vi "RTMain.Initialize.vi"(11 "Device Reference in":T1 format="%.0x") -> (0 "error out":errorcluster, 2 "Name":string, 3 "Parameters":T2 {"Settings"."Data Refs"."Write Refs" format="%.0x"; "Settings"."Data Refs"."Read Refs" format="%.0x"; "Settings"."Write Locations"."DataType" items=["Boolean"=1, "SByte"=2, "Byte"=3, "Int16"=4, "UInt16"=5, "Int32"=6, "UInt32"=7, "Int64"=8, "UInt64"=9, "Float"=10, "Double"=11, "String"=12, "DateTime"=13, "ByteString"=15, "Array of Boolean"=101, "Array of SByte"=102, "Array of Byte"=103, "Array of Int16"=104, "Array of UInt16"=105, "Array of Int32"=106, "Array of UInt32"=107, "Array of Int64"=108, "Array of UInt64"=109, "Array of Float"=110, "Array of Double"=111, "Array of String"=112, "Array of DateTime"=113, "Array of ByteString"=115]; "Settings"."StatusRefs"."Chan Refs" format="%.0x"})   [LabVIEW 2013, in "OPC UA Client Engine.lvlib"]
uses:
  OPC UA Client Engine.lvlib
  Types/PollEngine.Parameters.ctl
  Shared/Compiled.Settings.ctl
  Shared/Connection.Properties.ctl
  Shared/PollEngine.Settings.ctl
  <vilib>/NI Veristand/Custom Device API/Data Reference.ctl
  Shared/WriteData.Info.ctl
  Shared/ReadWriteRefs.ctl
  <vilib>/NI Veristand/Custom Device API/Custom Device Item Ref.ctl
  <vilib>/NI Veristand/Custom Device API/Get Item Property (Variant).vi
  Shared/Constants.vi
  <vilib>/NI Veristand/Custom Device API/Custom Device API.lvlib
  Shared/OPC UA Client Shared.lvlib
  <vilib>/OPCUA/NI OPC UA Client.lvlib
  <vilib>/NI VeriStand/Custom Device Tools/Custom Device Utility Library/Custom Device Utility Library.lvlib
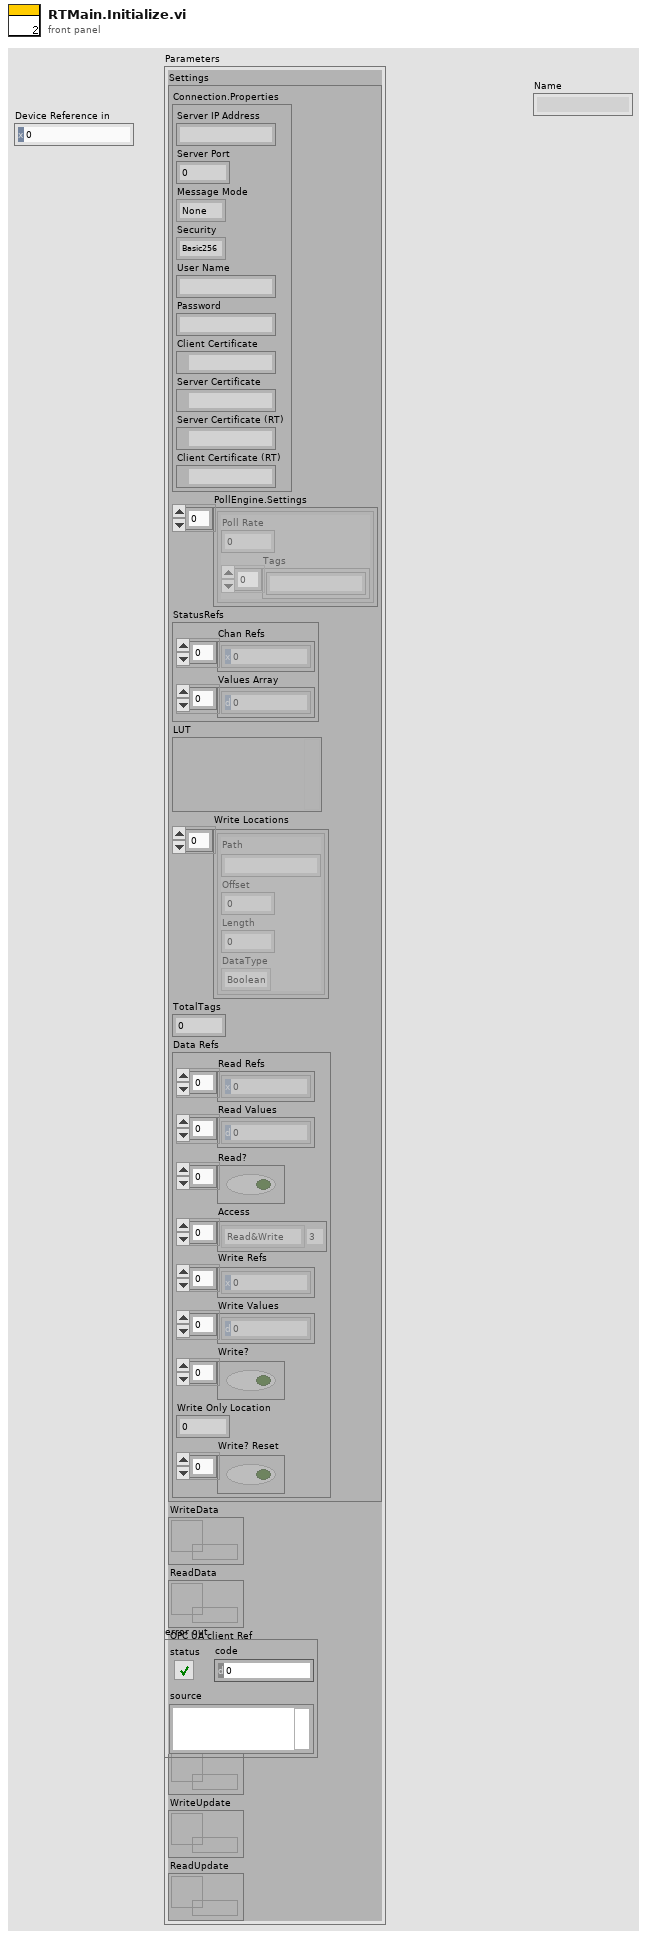
[diagram p1: front panel]
types:
  T1 = typedef "Custom Device API.lvlib/Custom Device Item Ref.ctl" = u64
  T2 = typedef "OPC UA Client Engine.lvlib/PollEngine.Parameters.ctl" = cluster{"Settings":T3, "WriteData":refnum<k33>, "ReadData":refnum<k33>, "OPC UA client Ref":refnum<k21>, "Data Change":refnum<user-event>, "StatusData":refnum<k33>, "WriteUpdate":refnum<k33>, "ReadUpdate":refnum<k33>}
  T3 = typedef "OPC UA Client Shared.lvlib/Compiled.Settings.ctl" = cluster{"Connection.Properties":T4, "PollEngine.Settings":T5[], "StatusRefs":cluster{"Chan Refs":T6[], "Values Array":dbl[]}, "LUT":variant, "Write Locations":T7[], "TotalTags":u32, "Data Refs":T8}
  T4 = typedef "OPC UA Client Shared.lvlib/Connection.Properties.ctl" = cluster{"Server IP Address":string, "Server Port":u16, "Message Mode":enum16{"None", "Sign", "Sign and Encrypt"}, "Security":enum16{"Basic256", "Basic128Rsa15"}, "User Name":string, "Password":string, "Client Certificate":path, "Server Certificate":path, "Server Certificate (RT)":path, "Client Certificate (RT)":path}
  T5 = typedef "OPC UA Client Shared.lvlib/PollEngine.Settings.ctl" = cluster{"Poll Rate":dbl, "Tags":string[]}
  T6 = typedef "Custom Device API.lvlib/Data Reference.ctl" = i32
  T7 = typedef "OPC UA Client Shared.lvlib/WriteData.Info.ctl" = cluster{"Path":string, "Offset":i32, "Length":i32, "DataType":u32}
  T8 = typedef "OPC UA Client Shared.lvlib/ReadWriteRefs.ctl" = cluster{"Read Refs":T6[], "Read Values":dbl[], "Read?":bool[], "Access":enum8{"Null", "Read", "Write", "Read&Write"}[], "Write Refs":T6[], "Write Values":dbl[], "Write?":bool[], "Write Only Location":u32, "Write? Reset":bool[]}
  T9 = cluster{"read mode":enum16{"polling", "blocking"}, "write mode":enum16{"polling", "blocking"}}
  T10 = cluster{"message mode":enum16{"None", "Sign", "Sign and Encrypt"}, "security":enum16{"Basic256", "Basic128Rsa15"}}
  T11 = typedef "Custom Device API.lvlib/Custom Device Item Info.ctl" = cluster{"Name":string, "Is Channel":bool, "GUID":string, "Is Waveform":bool}
  T12 = typedef "Custom Device API.lvlib/Custom Device Target Type.ctl" = enum16{"PharLap", "VxWorks", "Windows"}
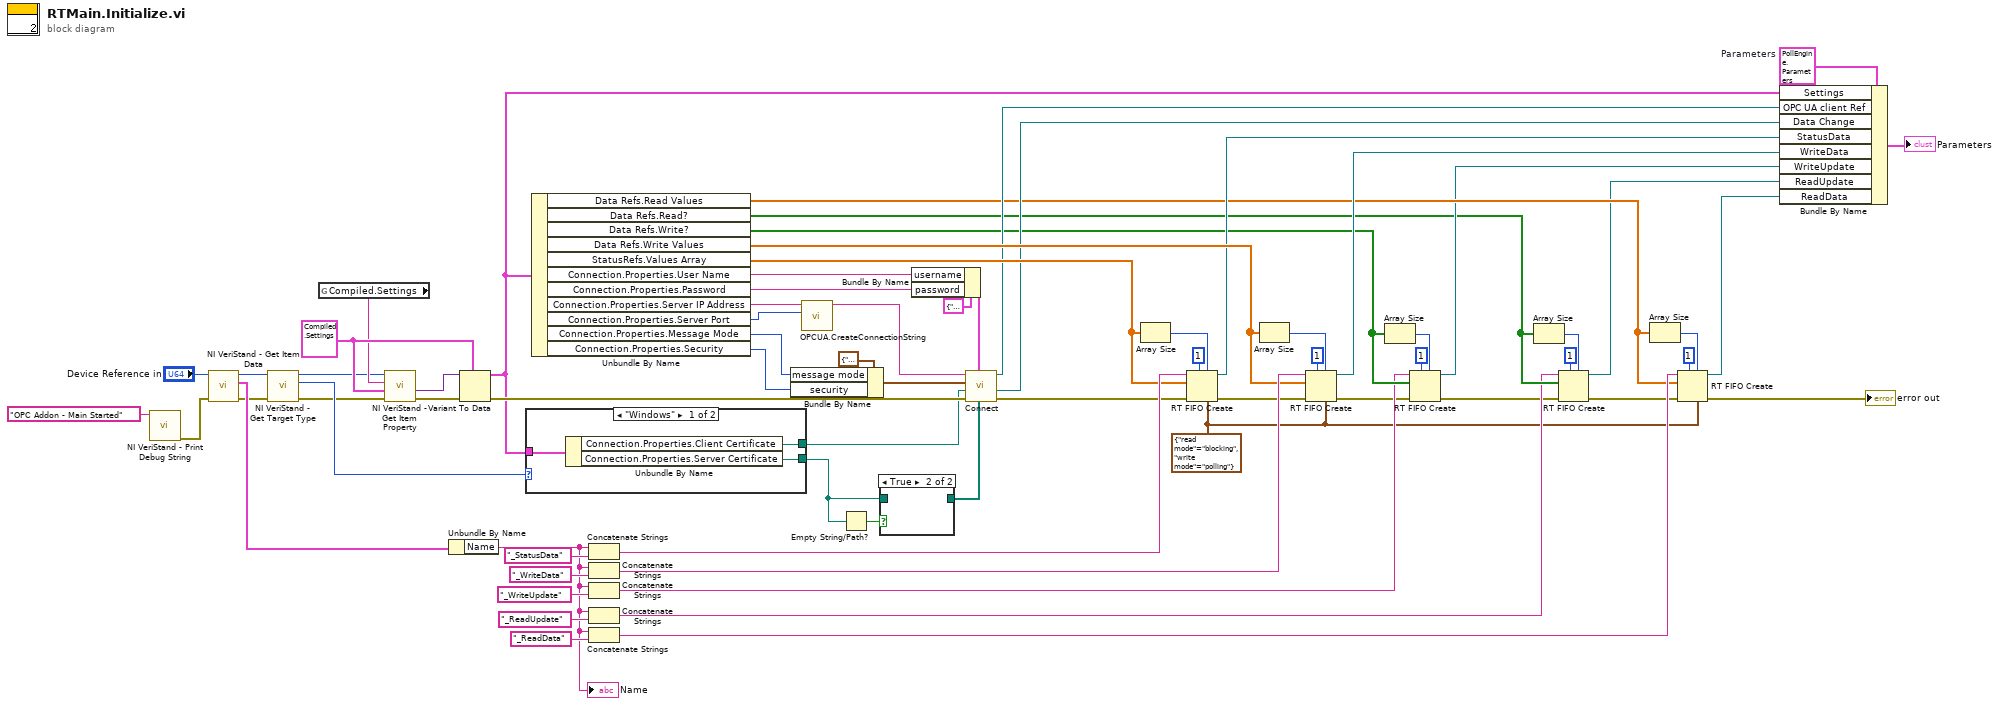
[diagram p0: block diagram]
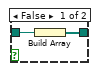
[diagram p2: hidden frame]
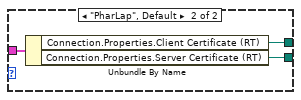
[diagram p3: hidden frame]
diagram:
  w12 = T9 {"read mode"=enum."blocking", "write mode"=enum."polling"} ("r/w modes (polling,polling)")
  w70 = T2 {"Settings"={"Connection.Properties"={"Server IP Address"="", "Server Port"=0, "Message Mode"=enum."None", "Security"=enum."Basic256", "User Name"="", "Password"="", "Client Certificate"=path "", "Server Certificate"=path "", "Server Certificate (RT)"=path "", "Client Certificate (RT)"=path ""}, "PollEngine.Settings"=[], "StatusRefs"={"Chan Refs"=[], "Values Array"=[]}, "LUT"=variant, "Write Locations"=[], "TotalTags"=0, "Data Refs"={"Read Refs"=[], "Read Values"=[], "Read?"=[], "Access"=[], "Write Refs"=[], "Write Values"=[], "Write?"=[], "Write Only Location"=0, "Write? Reset"=[]}}, "WriteData"=refnum, "ReadData"=refnum, "OPC UA client Ref"="", "Data Change"=refnum, "StatusData"=refnum, "WriteUpdate"=refnum, "ReadUpdate"=refnum}  # Parameters
  w63 = T3 {"Connection.Properties"={"Server IP Address"="", "Server Port"=0, "Message Mode"=enum."None", "Security"=enum."Basic256", "User Name"="", "Password"="", "Client Certificate"=path "", "Server Certificate"=path "", "Server Certificate (RT)"=path "", "Client Certificate (RT)"=path ""}, "PollEngine.Settings"=[], "StatusRefs"={"Chan Refs"=[], "Values Array"=[]}, "LUT"=variant, "Write Locations"=[], "TotalTags"=0, "Data Refs"={"Read Refs"=[], "Read Values"=[], "Read?"=[], "Access"=[], "Write Refs"=[], "Write Values"=[], "Write?"=[], "Write Only Location"=0, "Write? Reset"=[]}} ("Compiled.Settings")
  n1 = call <vilib>:"NI VeriStand - Print Debug String.vi"("Message"="OPC Addon - Main Started") -> ("error out"=w25:errorcluster)  [unwired: 10 in]
  n2 = call <vilib>:"NI VeriStand - Get Item Data.vi"("error in (no error)"=w25, "Item Ref in"="Device Reference in") -> ("error out"=w2:errorcluster, "Item Info"=w64:T11, "Item Ref out"=w1:T1)  [unwired: 6 in, 1 out]
  n3 = call <vilib>:"NI VeriStand - Get Target Type.vi"("error in (no error)"=w2, "Item Ref in"=w1) -> ("error out"=w41:errorcluster, "Target Type"=w44:T12, "Item Ref out"=w40:T1)  [unwired: 7 in]
  n4 = global read "Constants.vi" "Compiled.Settings"() -> (w62:string)
  n5 = call-poly <vilib>:"NI VeriStand - Get Item Property.vi"("error in (no error)"=w41, "Default Value"=w63, "Property Name"=w62, "Item Ref in"=w40) -> ("error out"=w60:errorcluster, "Value"=w61:variant)  [unwired: 4 in, 2 out]
  n6 = Unbundle By Name(w64) -> ("Name"=w31:string)
  "Name" <- w31
  n7 = Variant To Data(error in=w60, type=w63, Variant=w61) -> (data=w43:T3, error out=w48:errorcluster)
  n8 = case shown="\"Windows\"" w44 {
    tunnel: [w75 w78] -> w19
    tunnel: [w74 w77] -> w28
    tunnel: w43 -> [w73 w76]
    frame "Windows" {
      n9 = Unbundle By Name(w73) -> ("Connection.Properties.Client Certificate"=w75:path, "Connection.Properties.Server Certificate"=w74:path)
    }
    frame "PharLap", Default {
      n10 = Unbundle By Name(w76) -> ("Connection.Properties.Client Certificate (RT)"=w78:path, "Connection.Properties.Server Certificate (RT)"=w77:path)
    }
  }
  n11 = Unbundle By Name(w43) -> ("Data Refs.Read Values"=w39:dbl[], "Data Refs.Read?"=w33:bool[], "Data Refs.Write?"=w37:bool[], "Data Refs.Write Values"=w59:dbl[], "StatusRefs.Values Array"=w56:dbl[], "Connection.Properties.User Name"=w23:string, "Connection.Properties.Password"=w22:string, "Connection.Properties.Server IP Address"=w50:string, "Connection.Properties.Server Port"=w49:u16, "Connection.Properties.Message Mode"=w21:enum16{"None", "Sign", "Sign and Encrypt"}, "Connection.Properties.Security"=w20:enum16{"Basic256", "Basic128Rsa15"})
  n12 = Concatenate Strings(w31, "_StatusData" ("string")) -> (w57:string)
  n13 = Concatenate Strings(w31, "_WriteData" ("string")) -> (w67:string)
  n14 = Concatenate Strings(w31, "_WriteUpdate" ("string")) -> (w34:string)
  n15 = Concatenate Strings(w31, "_ReadUpdate" ("string")) -> (w30:string)
  n16 = Concatenate Strings(w31, "_ReadData" ("string")) -> (w68:string)
  n17 = Bundle By Name(cluster=T10 {"message mode"=enum."Sign", "security"=enum."Basic256"} ("security policy"), "message mode"=w21, "security"=w20) -> (w51:T10)
  n18 = call "OPCUA.CreateConnectionString.vi"("Server Port"=w49, "Server IP Address"=w50) -> ("concatenated string"=w24:string)  [unwired: 9 in]
  n19 = Empty String/Path?(string/path=w28) -> (empty?=w18:bool)
  n20 = case shown="True" w18 {
    tunnel: [w80 _] -> w27
    tunnel: w28 -> [w79 _]
    frame False {
      n21 = Build Array(w79) -> (w80:path[])
    }
    frame True {
    }
  }
  n22 = Bundle By Name(cluster=cluster{"username":string, "password":string} {"username"="", "password"=""} ("username/password"), "username"=w23, "password"=w22) -> (w53:cluster{"username":string, "password":string})
  n23 = call <vilib>:"Connect.vi"("trusted server certificates"=w27, "username/password"=w53, "error in (no error)"=w48, "client certificate file"=w19, "security policy"=w51, "server endpoint URL"=w24) -> ("error out"=w47:errorcluster, "OPC UA data change event"=w45:refnum<user-event>, "OPC UA client refnum out"=w46:refnum<k21>)  [unwired: 3 in]
  n24 = Array Size(array=w56) -> (size(s)=w15:i32)
  n25 = RT FIFO Create(0:w57, 1:w56, 3:w47, 4:u32 1 ("size (10)"), 6:w15, 7:w12) -> (8:w55:refnum<k33>, 11:w13:errorcluster)  [unwired: 2 in, 1 out]
  n26 = Array Size(array=w59) -> (size(s)=w16:i32)
  n27 = RT FIFO Create(0:w67, 1:w59, 3:w13, 4:u32 1 ("size (10)"), 6:w16, 7:w12) -> (8:w71:refnum<k33>, 11:w9:errorcluster)  [unwired: 2 in, 1 out]
  n28 = Array Size(array=w37) -> (size(s)=w8:i32)
  n29 = RT FIFO Create(0:w34, 1:w37, 3:w9, 4:u32 1 ("size (10)"), 6:w8) -> (8:w36:refnum<k33>, 11:w3:errorcluster)  [unwired: 3 in, 1 out]
  n30 = Array Size(array=w33) -> (size(s)=w5:i32)
  n31 = RT FIFO Create(0:w30, 1:w33, 3:w3, 4:u32 1 ("size (10)"), 6:w5) -> (8:w29:refnum<k33>, 11:w4:errorcluster)  [unwired: 3 in, 1 out]
  n32 = Array Size(array=w39) -> (size(s)=w11:i32)
  n33 = RT FIFO Create(0:w68, 1:w39, 3:w4, 4:u32 1 ("size (10)"), 6:w11, 7:w12) -> (8:w38:refnum<k33>, 11:→"error out":errorcluster)  [unwired: 2 in, 1 out]
  n34 = Bundle By Name(cluster=w70, "Settings"=w43, "OPC UA client Ref"=w46, "Data Change"=w45, "StatusData"=w55, "WriteData"=w71, "WriteUpdate"=w36, "ReadUpdate"=w29, "ReadData"=w38) -> (→"Parameters":T2)
